vi "DAC_example.vi"() -> ()   [LabVIEW 2012]
doc: "Equipment Required: This example expects a 34951 DAC card in slot 1 and a multiplexer card ( 34921 - 34925) in slot 2.\n\nThe example defines a trace named \"Example Trace\" on the 34951 DAC card and specifies it\nto be a sine wave. It then outputs that trace. The output of the DAC card is assumed to be wired into channel 2505 of a mulitplexer card in slot 2. The closing of channels 2005 and 2921 routes the signal to the 34980A's DMM.\n\nThe DMM then measures the DAC signal for AC Voltage and Frequency and the results are displayed."
panel:
  in  "VISA resource name":refnum<visa-resource-name>
  out "ACV Result":dbl[](array[numeric]) format="%.2e"
  out "Frequency Result":dbl[](array[numeric]) format="%.2e"
  out "VISA/Instrument Errors":errorcluster
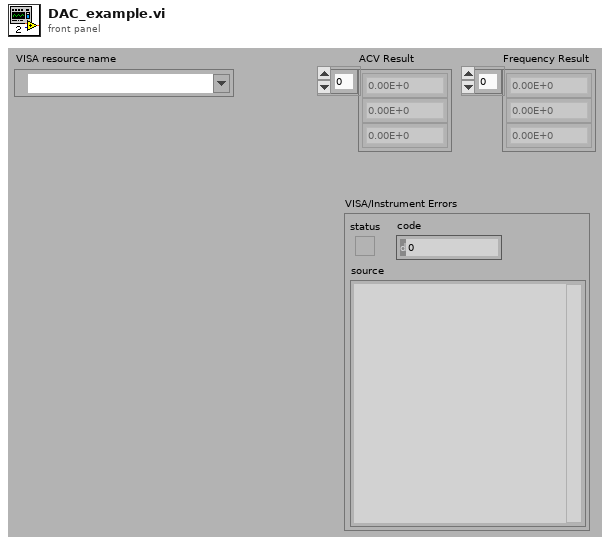
[diagram p1: front panel]
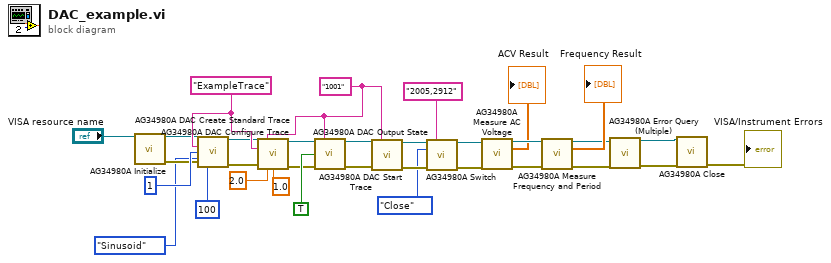
[diagram p0: block diagram]
diagram:
  w19 = "1001"
  w28 = "ExampleTrace"
  n1 = call "AG34980A Initialize.vi"("VISA resource name"="VISA resource name") -> ("VISA session"=w27:refnum<visa-resource-name>, "error out"=w26:errorcluster)  [unwired: 13 in]
  n2 = call "AG34980A DAC Create Standard Trace.vi"("VISA resource name"=w27, "Trace Name"=w28, "Slot (1)"=1, "Trace Type"=enum16{"Ramp", "Sinusoid", "Square", "Triangle"}."Sinusoid", "error in (no error)"=w26, "Num Points (1000)"=100) -> ("VISA resource name out"=w25:refnum<visa-resource-name>, "error out"=w24:errorcluster)  [unwired: 8 in]
  n3 = call "AG34980A DAC Configure Trace.vi"("VISA resource name"=w25, "Channel List"=w19, "Trace Name"=w28, "error in (no error)"=w24, "Gain (1)"=2.0, "Offset (0)"=1.0) -> ("VISA resource name out"=w23:refnum<visa-resource-name>, "error out"=w22:errorcluster)  [unwired: 8 in]
  n4 = call "AG34980A DAC Output State.vi"("VISA resource name"=w23, "Channel List"=w19, "Output State (F:Off)"=TRUE, "error in (no error)"=w22) -> ("VISA resource name out"=w21:refnum<visa-resource-name>, "error out"=w20:errorcluster)  [unwired: 10 in]
  n5 = call "AG34980A DAC Start Trace.vi"("VISA resource name"=w21, "Channel List"=w19, "error in (no error)"=w20) -> ("VISA resource name out"=w10:refnum<visa-resource-name>, "error out"=w9:errorcluster)  [unwired: 11 in]
  n6 = call "AG34980A Switch.vi"("VISA resource name"=w10, "Channel List"="2005,2912", "Open/Close (0:Close)"=enum16{"Close", "Open"}."Close", "error in (no error)"=w9) -> ("VISA resource name out"=w8:refnum<visa-resource-name>, "error out"=w7:errorcluster)  [unwired: 9 in, 1 out]
  n7 = call "AG34980A Measure AC Voltage.vi"("VISA resource name"=w8, "error in (no error)"=w7) -> ("VISA resource name out"=w15:refnum<visa-resource-name>, "Output Array"=→"ACV Result":dbl[], "error out"=w16:errorcluster)  [unwired: 11 in]
  n8 = call "AG34980A Measure Frequency and Period.vi"("VISA resource name"=w15, "error in (no error)"=w16) -> ("VISA resource name out"=w12:refnum<visa-resource-name>, "Output Array"=→"Frequency Result":dbl[], "error out"=w11:errorcluster)  [unwired: 11 in]
  n9 = call "AG34980A Error Query (Multiple).vi"("VISA resource name"=w12, "error in (no error)"=w11) -> ("VISA resource name out"=w17:refnum<visa-resource-name>, "error out"=w18:errorcluster)  [unwired: 10 in, 2 out]
  n10 = call "AG34980A Close.vi"("VISA resource name"=w17, "error in (no error)"=w18) -> ("error out"=→"VISA/Instrument Errors":errorcluster)  [unwired: 13 in]
